vi "MDAQ_Main.vi"() -> ()   [LabVIEW 2021]
uses:
  FunctionVIS/Status_Def.ctl
  FunctionVIS/GUI_Def.ctl
  FunctionVIS/Mode_Enum.ctl
  FunctionVIS/Status_Cluster.ctl
  FunctionVIS/Array_Cluster.ctl
  FunctionVIS/CMD_ARG_Enum.ctl
  FunctionVIS/ARG_Cluster.ctl
  <vilib>/Analysis/1siggen.llb/Ramp Pattern by Samples.vi
  <vilib>/Analysis/NI_AALBase.lvlib
panel:
  in  "Tab Control 2":T1(tab)
  out "MDAQ Monitor":string
  in  "Clear_Monitor_Button":bool
  in  "Print_Help_Button":bool
  in  "Load_Button":bool
  in  "Save_Button":bool
  in  "Clear_Button":bool
  out "Collecting":bool
  in  "StartAq_Button":bool
  out "Waveform Graph":u32[](graph)
  in  "Get_Button":bool
  in  "StopAq_Button":bool
  out "Progress":u8(slide) scale=0.0..30.0
  in  "ForceW_Button":bool
  in  "Tab Control 3":T2(tab)
  out "XY Graph":T3(graph)
  in  "Save_CV_Button":bool
  out "Temp Graph":T4(graph)
  in  "Save_CV_Button 2":bool
  out "Amplitude Plot":cluster{"X":dbl, "Y":dbl}[](graph)
  out "CurrectSpectrum":u32[](graph)
  out "Surface CV Plot":dbl[][](graph)
  out "Collecting CV":bool
  in  "StartCV_Button":bool
  in  "StopCV_Button":bool
  out "CV-Prog":u8(slide) scale=0.0..1.0
  in  "Tab Control 4":T5(tab)
  in  "Update_Cal_Button":bool
  in  "Stop":bool
  in  "Tab Control":T6(tab)
  out "Temp B (K)":dbl
  out "Temp A (K)":dbl
  in  "Call_LS335":bool
  in  "Reset_Button":bool
  in  "Channels":T7(radio)=enum."Item 1"
  in  "Wave Form":enum32{"Item 0", "Item 1", "Radio Selection 3"}(radio)=enum."Item 1"
  in  "Send_Button":bool
  in  "Gate Stop":dbl=87.5 min=0.0 max=100.0 format="%.1f%%"
  in  "Gate Start":dbl=12.5 min=0.0 max=100.0 format="%.1f%%"
  in  "Amplitude":dbl min=0.0 max=16383.0 step=1.0
  in  "Frequency":dbl=10.0 min=1.0 max=114.0 step=0.05 format="%.2g"
  out "LakeShore?":bool
  in  "User Comments":string="Enter Comments here!"
  in  "Sample Name":string="Default Name"
  in  "CV Mode":enum32{"Item 0", "Item 1"}(radio)
  out "Elapsed Time":dbl format="%<%H:%M>t"
  in  "Master File Path":path
  out "Current Scan No.":i32
  in  "SendRamp_Button":bool
  in  "Steps":dbl=1.0 min=1.0 max=16383.0 step=1.0 format="%#.0f"
  in  "End":dbl min=0.0 max=16383.0 step=1.0 format="%#.0f"
  in  "Start":dbl min=0.0 max=16383.0 step=1.0 format="%#.0f"
  in  "Normalise Graph":bool
  out "Current Index":u32
  out "Delta T per Cycle (s)":dbl
  out "Target Values":i32
  in  "Refresh CV":bool
  in  "Target Bins/Ampl":dbl[](array[numeric]) min=0.0 max=16383.0 step=1.0
  in  "Delta T (s)":dbl=30.0
  in  "Manual_Send":bool
  in  "String":string
  out "error out":errorcluster {"code" format="%.0x"}
  in  "MDAQ209B COM Port":refnum<visa-resource-name>="COM4"
  # "Regular"
  # "Mirror"
  # "Index 0 is the value used for normalisation"
  # "Min:  0\nZero: \nMax: 16383"
  # "WARNING! Only use this function if you understand how the text\ncommands of the MDAQ works. Failure to do so may freeze the MDAQ\nand require you to power cylce the device. You have been warned."
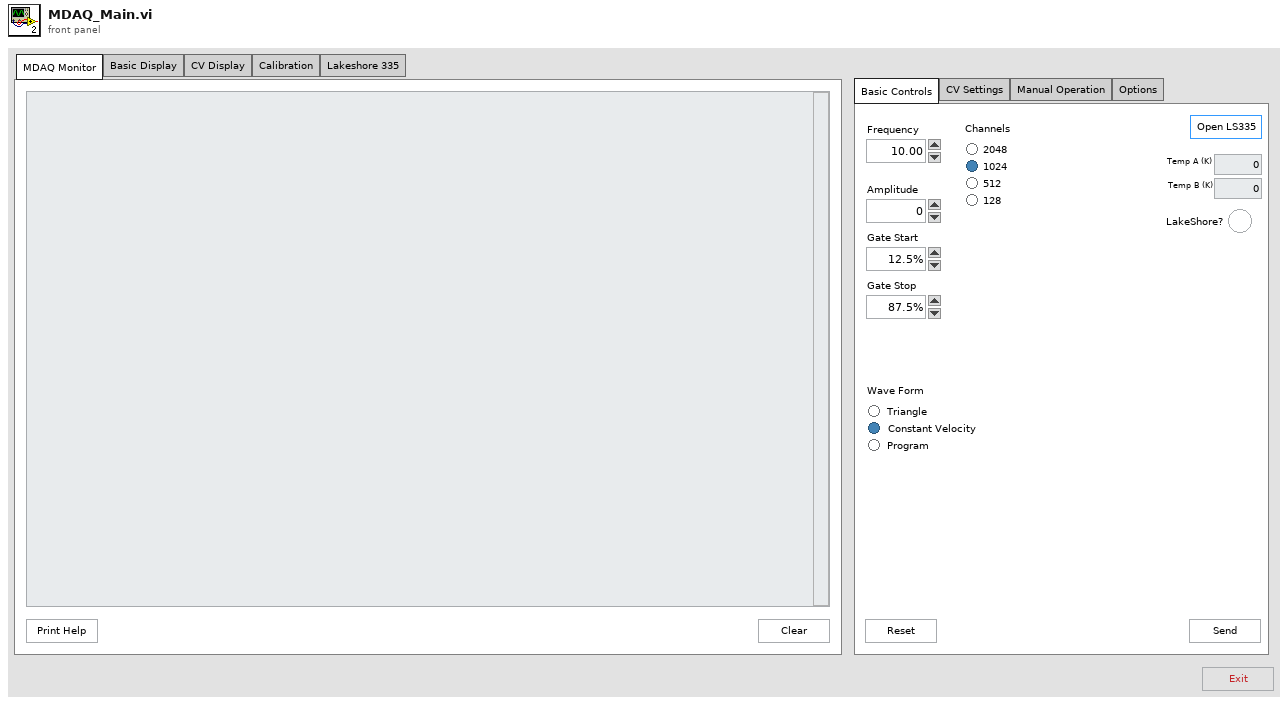
[diagram p1: front panel]
types:
  T1 = enum32{"MDAQ Monitor", "Basic Display", "CV Display", "Calibration", "Lakeshore 335"}
  T2 = enum32{"Time Plot", "Temperature Plot", "Amplitude Plot", "Current Spectrum", "Surface CV Plot"}
  T3 = cluster{"SetPointArray":cluster{timestamp, dbl}[]}[]
  T4 = cluster{"Counts Array":cluster{"Avg Temp":dbl, dbl}[]}[]
  T5 = enum32{"Spectrum Selection", "Calibration Overview"}
  T6 = enum32{"Basic Controls", "CV Settings", "Manual Operation", "Options"}
  T7 = enum32{"Item 0", "Item 1", "Radio Selection 3", ""}
  T8 = enum8{"Enabled", "Disabled", "Disabled and Grayed Out"}
  T9 = typedef "Status_Def.ctl" = enum16{"ClearCVCycle", "WriteCVData", "SendRamp", "LoadSpectrum", "RefreshCV", "SaveCVPlot", "GetCVSpectrum", "ConfigCV", "StopCV", "StartCV", "SaveSpectrum", "Clear Spectrum", "StopCollecting", "StopAq", "StartAq", "Reset MDAQ", "Get Spectrum", "Clear Monitor", "Idle", "String Send", "Settings Send", "Read Help"}
  T10 = typedef "Array_Cluster.ctl" = cluster{"CV Data Array":cluster{"Counts Array":cluster{timestamp, i32}[]}[], "CV Normalised Array":cluster{"Counts Array":cluster{timestamp, dbl}[]}[], "CV Temp Array":cluster{"Counts Array":cluster{"Avg Temp":dbl, dbl}[]}[]}
  T11 = typedef "Status_Cluster.ctl" = cluster{"CHAN":u32, "BASE":u32, "STEP":u32, "N_CYCLES":u32, "M_CYCLES":u32, "AMPLITUDE":u32, "GATESTRT":u32, "GATESTOP":u32, "Spectrum Array":u32[], "Spectrum Cycle":u32[][], "Cycle Timestamps":timestamp[], "Temperature Collect":dbl[]}
  T12 = typedef "GUI_Def.ctl" = cluster{"Monitor MSG":string, "Request Read":bool, "Cycle TimeStamp":timestamp, "CV":cluster{"Set Point Index":u32, "Run Start TimeS":timestamp, "Last SP Index":u32, "No. Set Points":u32, "Target Set Points":i32[], "Reverse?":bool, "NormalizationFactor":i32[], "CycleNo":i32, "SurfaceCV":dbl[][], "New Cycle":bool, "Temperature Array":dbl[][]}, "Normal":cluster{"Collecting":bool}, "Getting Mode":T13}
  T13 = typedef "Mode_Enum.ctl" = enum16{"Off", "Normal", "CV+Temp", "CV"}
  T14 = typedef "CMD_ARG_Enum.ctl" = enum16{"N_Cycles", "GateStep", "ASCII_Spectrum", "Waveform", "GateStop", "GateStart", "Amplitude", "Frequency"}
  T15 = typedef "ARG_Cluster.ctl" = cluster{"Freq":dbl, "Amp":dbl, "Chan Start":dbl, "Chan End":dbl, "Wave Form":enum32{"Item 0", "Item 1", "Radio Selection 3"}, "Channels":enum32{"Item 0", "Item 1", "Radio Selection 3", ""}}
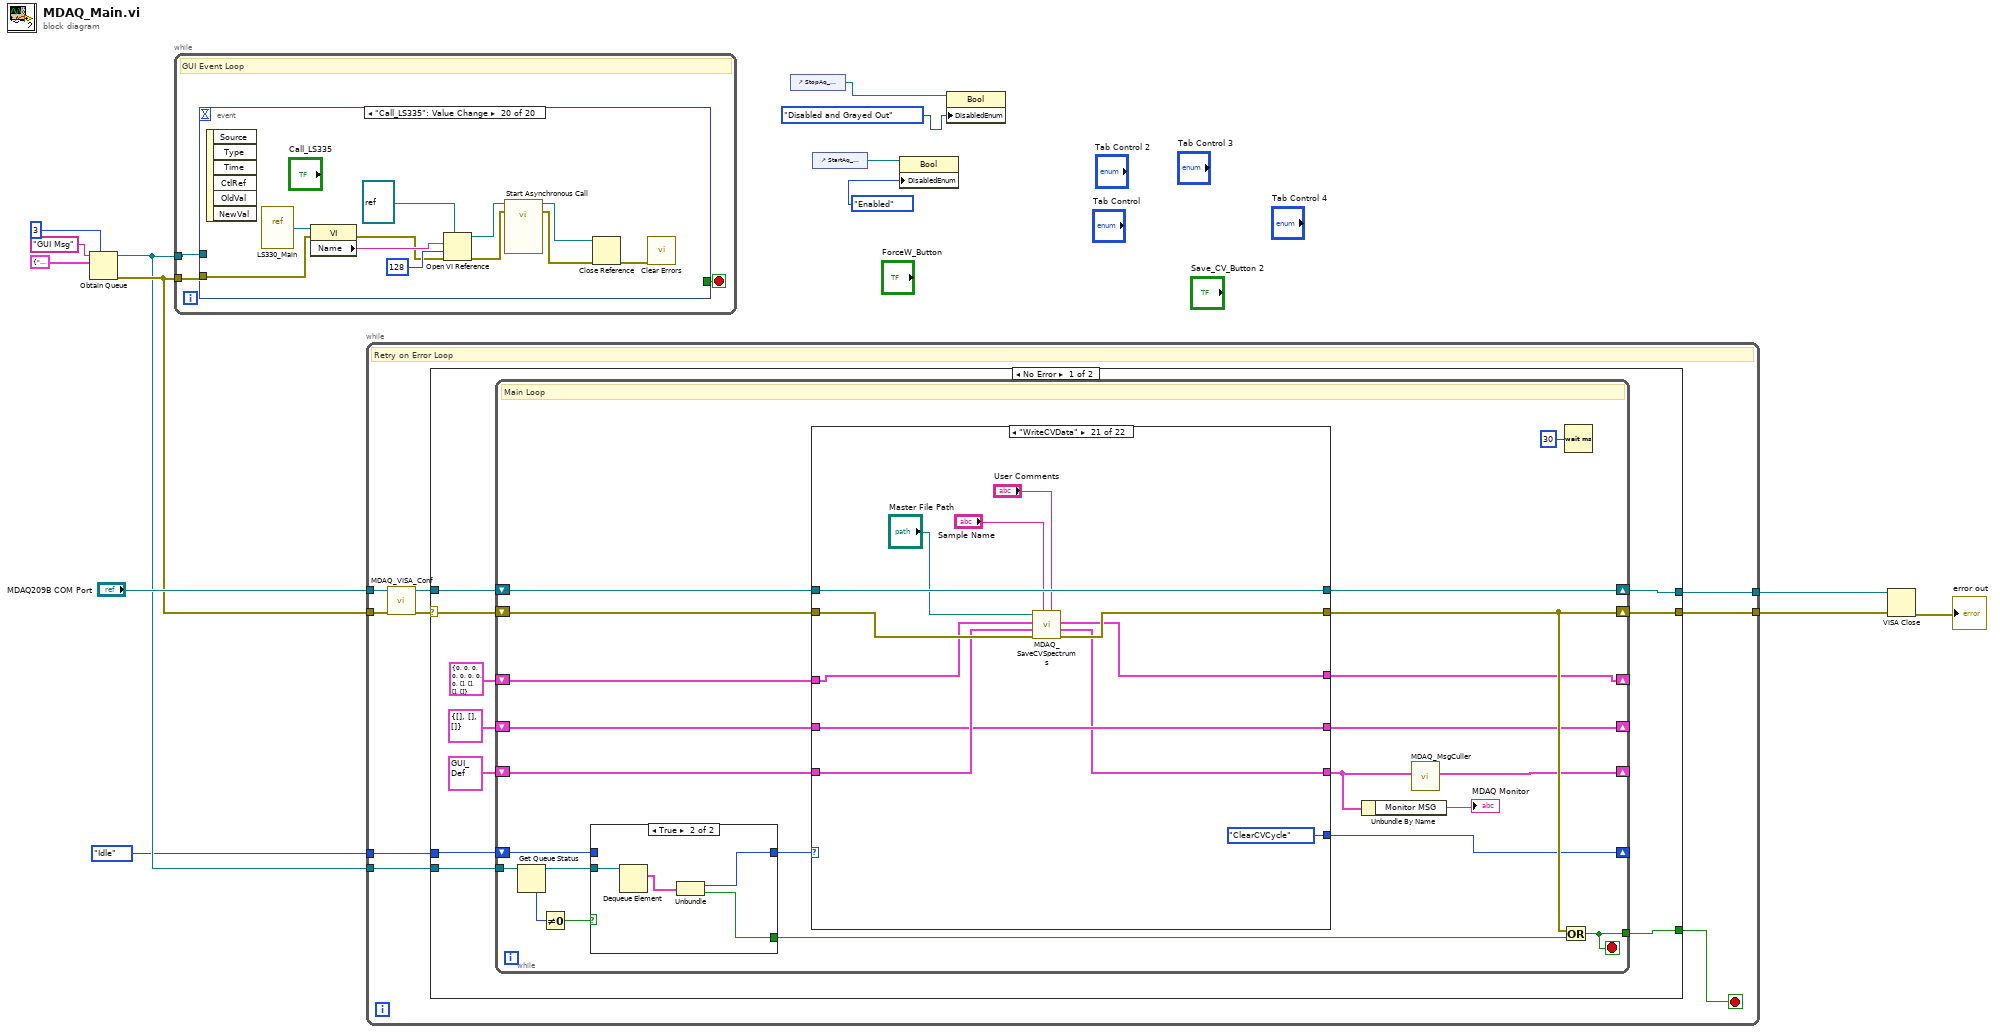
[diagram p0: block diagram]
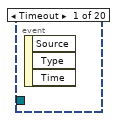
[diagram p2: hidden frame]
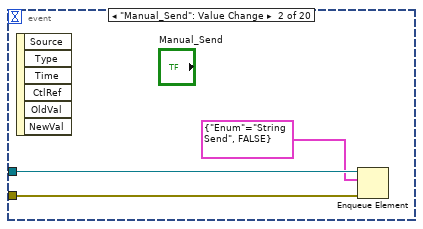
[diagram p3: hidden frame]
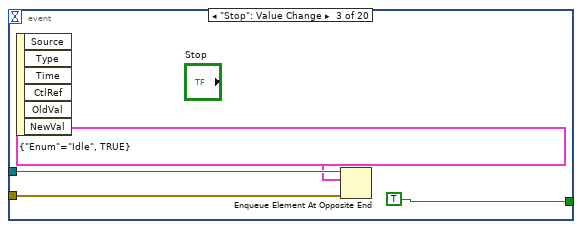
[diagram p4: hidden frame]
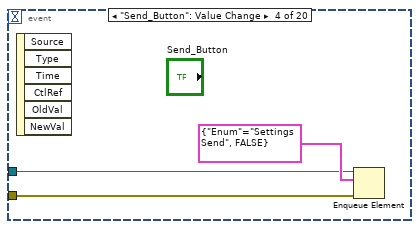
[diagram p5: hidden frame]
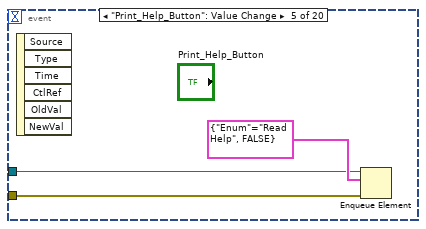
[diagram p6: hidden frame]
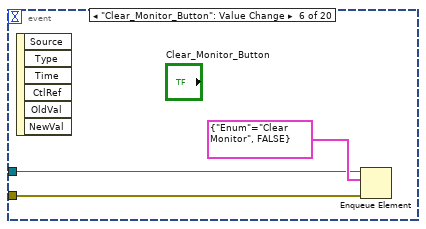
[diagram p7: hidden frame]
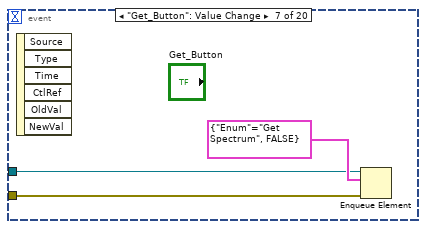
[diagram p8: hidden frame]
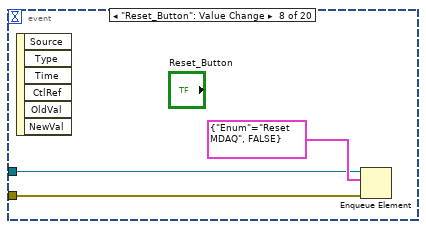
[diagram p9: hidden frame]
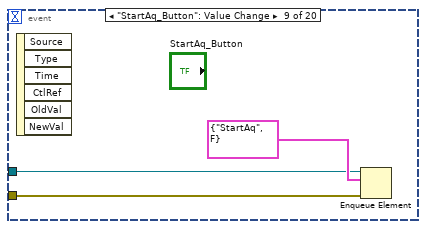
[diagram p10: hidden frame]
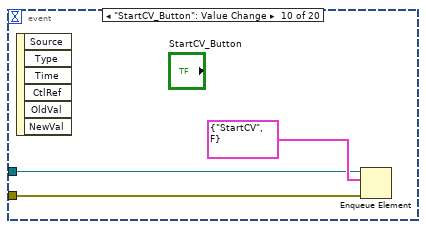
[diagram p11: hidden frame]
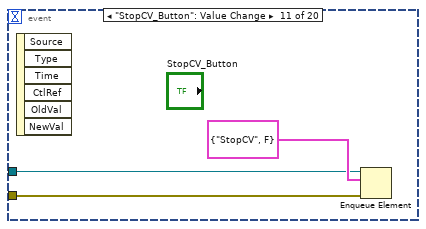
[diagram p12: hidden frame]
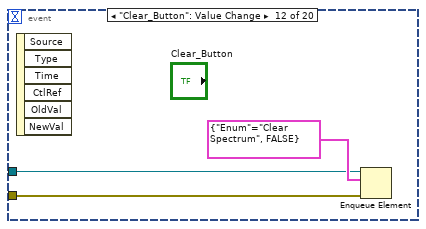
[diagram p13: hidden frame]
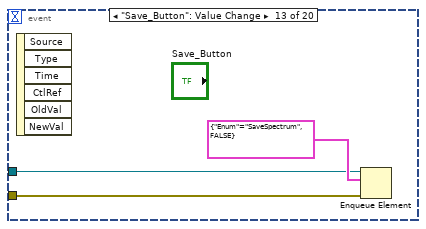
[diagram p14: hidden frame]
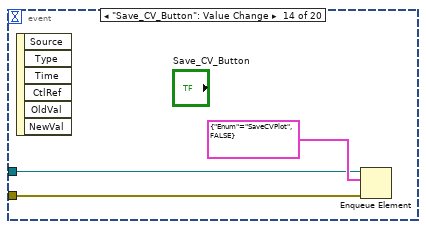
[diagram p15: hidden frame]
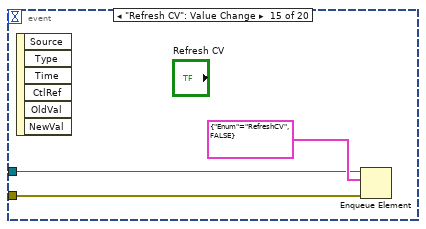
[diagram p16: hidden frame]
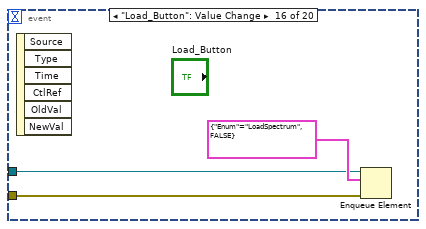
[diagram p17: hidden frame]
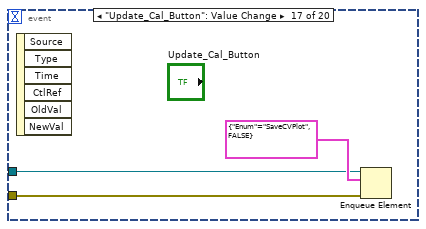
[diagram p18: hidden frame]
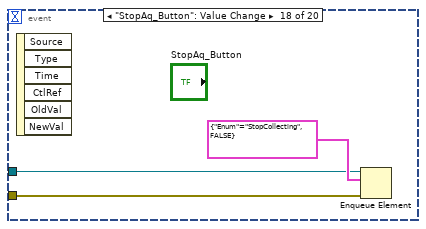
[diagram p19: hidden frame]
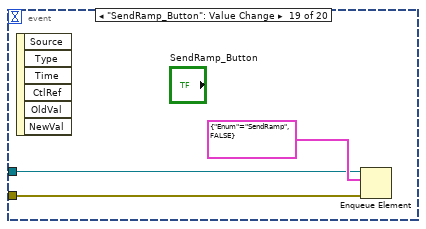
[diagram p20: hidden frame]
diagram:
  n1 = Obtain Queue(max queue size (-1, unlimited)=3, name (unnamed)="GUI Msg", element data type=cluster{"Enum":T9, bool} {"Enum"=enum."Read Help", TRUE}) -> (queue out=w9:refnum<queue>, error out=w10:errorcluster)  [unwired: 2 in, 1 out]
  n2 = while {
    tunnel: w10 -> [w17]
    tunnel: w9 -> [w16]
    stop <- w15 stop-if-true
    # "GUI Event Loop"
    n3 = event shown="[19] \"Call_LS335\": Value Change" {
      selector: _ -> [_ _ _ _ _ _ _ _ _ _ _ _ _ _ _ _ _ _ _ _]
      dyn-events: _ -> [_ _ _ _ _ _ _ _ _ _ _ _ _ _ _ _ _ _ _ _]
      timeout: _ -> [_ _ _ _ _ _ _ _ _ _ _ _ _ _ _ _ _ _ _ _]
      tunnel: w16 -> [_ w20 w24 w26 w29 w32 w35 w38 w41 w44 w47 w50 w53 w56 w59 w62 w65 w68 w71 _]
      tunnel: w17 -> [_ w18 w23 w25 w28 w31 w34 w37 w40 w43 w46 w49 w52 w55 w58 w61 w64 w67 w70 w80]
      tunnel: [_ _ TRUE _ _ _ _ _ _ _ _ _ _ _ _ _ _ _ _ _] -> w15
      event Timeout {
        n4 = event-data() -> ()  [unwired: 1 in, 3 out]
      }
      event "Manual_Send": Value Change {
        n5 = event-data() -> ()  [unwired: 1 in, 6 out]
        n6 = Enqueue Element(queue=w20, element=cluster{"Enum":T9, bool} {"Enum"=enum."String Send", FALSE}, error in (no error)=w18) -> ()  [unwired: 1 in, 3 out]
      }
      event "Stop": Value Change {
        n7 = event-data() -> ()  [unwired: 1 in, 6 out]
        n8 = Enqueue Element At Opposite End(queue=w24, element=cluster{"Enum":T9, bool} {"Enum"=enum."Idle", TRUE}, error in (no error)=w23) -> ()  [unwired: 1 in, 3 out]
      }
      event "Send_Button": Value Change {
        n9 = event-data() -> ()  [unwired: 1 in, 6 out]
        n10 = Enqueue Element(queue=w26, element=cluster{"Enum":T9, bool} {"Enum"=enum."Settings Send", FALSE}, error in (no error)=w25) -> ()  [unwired: 1 in, 3 out]
      }
      event "Print_Help_Button": Value Change {
        n11 = event-data() -> ()  [unwired: 1 in, 6 out]
        n12 = Enqueue Element(queue=w29, element=cluster{"Enum":T9, bool} {"Enum"=enum."Read Help", FALSE}, error in (no error)=w28) -> ()  [unwired: 1 in, 3 out]
      }
      event "Clear_Monitor_Button": Value Change {
        n13 = event-data() -> ()  [unwired: 1 in, 6 out]
        n14 = Enqueue Element(queue=w32, element=cluster{"Enum":T9, bool} {"Enum"=enum."Clear Monitor", FALSE}, error in (no error)=w31) -> ()  [unwired: 1 in, 3 out]
      }
      event "Get_Button": Value Change {
        n15 = event-data() -> ()  [unwired: 1 in, 6 out]
        n16 = Enqueue Element(queue=w35, element=cluster{"Enum":T9, bool} {"Enum"=enum."Get Spectrum", FALSE}, error in (no error)=w34) -> ()  [unwired: 1 in, 3 out]
      }
      event "Reset_Button": Value Change {
        n17 = event-data() -> ()  [unwired: 1 in, 6 out]
        n18 = Enqueue Element(queue=w38, element=cluster{"Enum":T9, bool} {"Enum"=enum."Reset MDAQ", FALSE}, error in (no error)=w37) -> ()  [unwired: 1 in, 3 out]
      }
      event "StartAq_Button": Value Change {
        n19 = event-data() -> ()  [unwired: 1 in, 6 out]
        n20 = Enqueue Element(queue=w41, element=cluster{"Enum":T9, bool} {"Enum"=enum."StartAq", FALSE}, error in (no error)=w40) -> ()  [unwired: 1 in, 3 out]
      }
      event "StartCV_Button": Value Change {
        n21 = event-data() -> ()  [unwired: 1 in, 6 out]
        n22 = Enqueue Element(queue=w44, element=cluster{"Enum":T9, bool} {"Enum"=enum."StartCV", FALSE}, error in (no error)=w43) -> ()  [unwired: 1 in, 3 out]
      }
      event "StopCV_Button": Value Change {
        n23 = event-data() -> ()  [unwired: 1 in, 6 out]
        n24 = Enqueue Element(queue=w47, element=cluster{"Enum":T9, bool} {"Enum"=enum."StopCV", FALSE}, error in (no error)=w46) -> ()  [unwired: 1 in, 3 out]
      }
      event "Clear_Button": Value Change {
        n25 = event-data() -> ()  [unwired: 1 in, 6 out]
        n26 = Enqueue Element(queue=w50, element=cluster{"Enum":T9, bool} {"Enum"=enum."Clear Spectrum", FALSE}, error in (no error)=w49) -> ()  [unwired: 1 in, 3 out]
      }
      event "Save_Button": Value Change {
        n27 = event-data() -> ()  [unwired: 1 in, 6 out]
        n28 = Enqueue Element(queue=w53, element=cluster{"Enum":T9, bool} {"Enum"=enum."SaveSpectrum", FALSE}, error in (no error)=w52) -> ()  [unwired: 1 in, 3 out]
      }
      event "Save_CV_Button": Value Change {
        n29 = event-data() -> ()  [unwired: 1 in, 6 out]
        n30 = Enqueue Element(queue=w56, element=cluster{"Enum":T9, bool} {"Enum"=enum."SaveCVPlot", FALSE}, error in (no error)=w55) -> ()  [unwired: 1 in, 3 out]
      }
      event "Refresh CV": Value Change {
        n31 = event-data() -> ()  [unwired: 1 in, 6 out]
        n32 = Enqueue Element(queue=w59, element=cluster{"Enum":T9, bool} {"Enum"=enum."RefreshCV", FALSE}, error in (no error)=w58) -> ()  [unwired: 1 in, 3 out]
      }
      event "Load_Button": Value Change {
        n33 = event-data() -> ()  [unwired: 1 in, 6 out]
        n34 = Enqueue Element(queue=w62, element=cluster{"Enum":T9, bool} {"Enum"=enum."LoadSpectrum", FALSE}, error in (no error)=w61) -> ()  [unwired: 1 in, 3 out]
      }
      event "Update_Cal_Button": Value Change {
        n35 = event-data() -> ()  [unwired: 1 in, 6 out]
        n36 = Enqueue Element(queue=w65, element=cluster{"Enum":T9, bool} {"Enum"=enum."SaveCVPlot", FALSE}, error in (no error)=w64) -> ()  [unwired: 1 in, 3 out]
      }
      event "StopAq_Button": Value Change {
        n37 = event-data() -> ()  [unwired: 1 in, 6 out]
        n38 = Enqueue Element(queue=w68, element=cluster{"Enum":T9, bool} {"Enum"=enum."StopCollecting", FALSE}, error in (no error)=w67) -> ()  [unwired: 1 in, 3 out]
      }
      event "SendRamp_Button": Value Change {
        n39 = event-data() -> ()  [unwired: 1 in, 6 out]
        n40 = Enqueue Element(queue=w71, element=cluster{"Enum":T9, bool} {"Enum"=enum."SendRamp", FALSE}, error in (no error)=w70) -> ()  [unwired: 1 in, 3 out]
      }
      event "Call_LS335": Value Change {
        n41 = event-data() -> ()  [unwired: 1 in, 6 out]
        n42 = vi-ref "LS330_Main.vi"() -> (w83:refnum<vi>)
        n43 = property class="VI"(reference=w83, error in=w80) -> (error out=w79:errorcluster, "Name"=w82:string)  [unwired: 1 out]
        n44 = Open VI Reference(type specifier VI Refnum (for type only)=refnum<vi> refnum, vi path=w82, options=128, error in (no error)=w79) -> (vi reference=w76:refnum<vi>, error out=w78:errorcluster)  [unwired: 2 in]
        n45 = call-by-ref "Start Asynchronous Call"(reference=w76, error in=w78) -> (reference out=w75:refnum<vi>, error out=w74:errorcluster)  [unwired: 12 in]
        n46 = Close Reference(reference=w75, error in (no error)=w74) -> (error out=w73:errorcluster)
        n47 = call <vilib>:"Clear Errors.vi"("error in (no error)"=w73) -> ()  [unwired: 5 in, 2 out]
      }
    }
  }
  n48 = while {
    tunnel: "MDAQ209B COM Port" -> [w92]
    tunnel: w10 -> [w90]
    tunnel: w9 -> [w88]
    tunnel: [w87] -> w7
    tunnel: [w86] -> w8
    tunnel: Status_Def."Idle" ("Enum") -> [w84]
    stop <- w85 stop-if-true
    # "Retry on Error Loop"
    n49 = call "MDAQ_VISA_Conf.vi"("error in"=w90, "VISA resource name"=w92) -> ("error out"=w91:errorcluster, "VISA resource name out"=w89:refnum<visa-resource-name>)  [unwired: 8 in]
    n50 = case shown="No Error" w91 {
      selector: w91 -> [w100 w596]
      tunnel: w89 -> [w101 w597]
      tunnel: w88 -> [w102 _]
      tunnel: [w99 w596] -> w87
      tunnel: [w98 w597] -> w86
      tunnel: [w97 TRUE] -> w85
      tunnel: w84 -> [w96 _]
      frame No Error {
        n51 = while {
          tunnel: w102 -> [w121]
          shift-right: [w117] -> w98
          shift-left: w101 -> [w119]
          shift-right: [w116] -> w99
          shift-left: w100 -> [w118]
          shift-right: [w103] -> _
          shift-left: T12 {"Monitor MSG"="", "Request Read"=FALSE, "Cycle TimeStamp"=timestamp(0 s since 1904-01-01), "CV"={"Set Point Index"=0, "Run Start TimeS"=timestamp(0 s since 1904-01-01), "Last SP Index"=0, "No. Set Points"=0, "Target Set Points"=[], "Reverse?"=FALSE, "NormalizationFactor"=[], "CycleNo"=0, "SurfaceCV"=[], "New Cycle"=FALSE, "Temperature Array"=[]}, "Normal"={"Collecting"=FALSE}, "Getting Mode"=enum."Off"} ("Main Cluster") -> [w110]
          tunnel: [w114] -> w97
          shift-right: [w111] -> _
          shift-left: w96 -> [w112]
          shift-right: [w107] -> _
          shift-left: T11 {"CHAN"=0, "BASE"=0, "STEP"=0, "N_CYCLES"=0, "M_CYCLES"=0, "AMPLITUDE"=0, "GATESTRT"=0, "GATESTOP"=0, "Spectrum Array"=[], "Spectrum Cycle"=[], "Cycle Timestamps"=[], "Temperature Collect"=[]} ("Status Cluster") -> [w108]
          shift-right: [w106] -> _
          shift-left: T10 {"CV Data Array"=[], "CV Normalised Array"=[], "CV Temp Array"=[]} ("Concurrent CV Arrays") -> [w105]
          stop <- w114 stop-if-true
          # "Main Loop"
          n52 = Get Queue Status(queue=w121) -> (queue out=w122:refnum<queue>, # elements in queue=w123:i32)  [unwired: 2 in, 6 out]
          n53 = Not Equal To 0?(x=w123) -> (x != 0?=w124:bool)
          n54 = case shown="True" w124 {
            tunnel: w122 -> [_ w130]
            tunnel: w112 -> [w126 _]
            tunnel: [w126 w128] -> w120
            tunnel: [FALSE w127] -> w115
            frame False {
            }
            frame True {
              n55 = Dequeue Element(queue=w130) -> (element=w129:cluster{"Enum":T9, bool})  [unwired: 2 in, 3 out]
              n56 = Unbundle(w129) -> ("Enum"=w128:T9, w127:bool)
            }
          }
          n57 = case shown="\"WriteCVData\"" w120 {
            selector: w120 -> [w139 _ _ _ _ _ _ _ _ _ _ _ _ _ _ _ _ _ _ _ _ _]
            tunnel: [w136 Status_Def."Idle" ("Enum") Status_Def."Idle" ("Enum") w221 Status_Def."Idle" ("Enum") Status_Def."ConfigCV" ("Enum") Status_Def."Idle" ("Enum") w327 Status_Def."Idle" ("Enum") Status_Def."Idle" ("Enum") w384 w429 Status_Def."Idle" ("Enum") Status_Def."Idle" ("Enum") Status_Def."Idle" ("Enum") Status_Def."Idle" ("Enum") w524 w545 Status_Def."Idle" ("Enum") Status_Def."Idle" ("Enum") Status_Def."ClearCVCycle" ("Enum") Status_Def."Idle" ("Enum")] -> w111
            tunnel: w119 -> [w146 w201 w212 w233 w247 w283 w312 w340 w355 w360 w382 w435 w476 w488 w492 w501 w536 w543 w561 w567 w580 w588]
            tunnel: w118 -> [w145 w200 w211 w232 w246 w282 w311 w337 w354 w359 w381 w434 w458 w487 w491 w499 w535 w542 w557 w563 w577 w587]
            tunnel: [w148 w197 w208 w231 w248 w280 w309 w342 w354 w357 w379 w423 w457 w486 w491 w504 w527 w544 w556 w565 w574 w587] -> w116
            tunnel: [w147 w198 w209 w230 w249 w281 w310 w343 w355 w358 w380 w424 w476 w485 w492 w505 w528 w543 w561 w567 w580 w588] -> w117
            tunnel: [w142 w204 w216 w228 w259 w267 w302 w322 w352 w370 w385 w406 w462 w481 w494 w514 w533 w551 w560 w564 w571 w584] -> w104
            tunnel: w110 -> [w135 w206 w218 w229 w261 w289 w301 w331 w352 w372 w376 w427 w467 w483 w496 w515 w526 w549 w560 w564 w575 w585]
            tunnel: w108 -> [w133 w203 w215 w227 w258 w273 w299 w339 w353 w369 w378 w433 w475 w480 w493 w500 w534 w541 w558 w566 w576 w583]
            tunnel: [w132 w203 w215 w227 w258 w272 w299 w324 w353 w369 w377 w407 w475 w480 w493 w503 w519 w541 w555 w566 w572 w582] -> w107
            tunnel: [w131 w202 w214 w220 w250 w266 w293 w313 w345 w356 w374 w401 w456 w478 w489 w498 w517 w539 w552 w562 w573 w581] -> w106
            tunnel: w105 -> [w131 w202 w214 w220 w250 w265 w293 w313 w345 w356 w374 w402 w456 w478 w489 w498 w517 w539 w552 w562 w573 w581]
            frame "Idle", Default {
              n58 = Unbundle By Name(w135) -> ("Monitor MSG"=w144:string, "Request Read"=w143:bool, "Cycle TimeStamp"=w137:timestamp, "Getting Mode"=w138:T13)
              n59 = case shown="False" w143 {
                tunnel: w145 -> [w186 w194]
                tunnel: [w186 w192] -> w148
                tunnel: [w187 w193] -> w147
                tunnel: w146 -> [w187 w195]
                tunnel: [FALSE w191] -> w141
                tunnel: w144 -> [w184 w190]
                tunnel: [w184 w188] -> w140
                frame False {
                }
                frame True {
                  n60 = call "MDAQ_ReadAll.vi"("error in"=w194, "VISA resource name"=w195) -> ("error IO"=w192:errorcluster, "Buffer Not Empty"=w191:bool, "read buffer"=w189:string, "VISA resource name out"=w193:refnum<visa-resource-name>)  [unwired: 6 in]
                  n61 = Concatenate Strings(w190, w189) -> (w188:string)
                }
              }
              n62 = case shown="\"CV+Temp\"" w138 {
                tunnel: w139 -> [w150 w158 w168 w179]
                tunnel: w137 -> [_ w161 _ _]
                tunnel: [w150 w154 w164 w178] -> w136
                tunnel: w135 -> [w151 w153 w167 w180]
                tunnel: [w151 w153 w166 w177] -> w134
                tunnel: w133 -> [w149 w152 w163 w176]
                tunnel: [w149 w152 w163 w175] -> w132
                frame "Off", Default {
                }
                frame "Normal" {
                  (unwired) 0.0
                  n63 = Get Date/Time In Seconds() -> (seconds since 1Jan1904=w162:timestamp)
                  n64 = Subtract(x=w162, y=w161) -> (x-y=w155:dbl)
                  n65 = Greater Or Equal?(x=w155, y=30.0) -> (x >= y?=w159:bool)
                  n66 = To Unsigned Byte Integer(number=w155) -> (unsigned 8bit integer=→"Progress":u8)
                  n67 = Select(t=Status_Def."StopAq", s=w159, f=w158) -> (s? t:f=w154:T9)
                }
                frame "CV" {
                  # "Idle"
                  # "StopAq"
                  n68 = control-ref of="CV-Prog"() -> (w171:refnum<vi>)
                  n69 = call "MDAQ_KeepTime.vi"("Delta T (s)"="Delta T (s)", "State in"=w168, "Cluster In"=w167, "Slide in"=w171) -> ("State Out"=w164:T9, "Cluster Out"=w166:T12, "Progress"=→"CV-Prog":u8, "Elapsed Out"=→"Elapsed Time":dbl)  [unwired: 4 in]
                }
                frame "CV+Temp" {
                  # "Idle"
                  # "StopAq?"
                  n70 = control-ref of="Elapsed Time"() -> (w181:refnum<vi>)
                  n71 = control-ref of="CV-Prog"() -> (w183:refnum<vi>)
                  n72 = control-ref of="Delta T (s)"() -> (w182:refnum<vi>)
                  n73 = call "MDAQ_GetTimeTemp.vi"("Elapsed Time Ref"=w181, "Delta T (s) Ref"=w182, "State in"=w179, "Cluster In"=w180, "Status In"=w176, "CV-Prog Ref"=w183) -> ("State Out"=w178:T9, "Cluster Out"=w177:T12, "Status Out"=w175:T11, "Temps"=w174:cluster{"Double":dbl, "Double":dbl})  [unwired: 2 in]
                  n74 = Unbundle(w174) -> ("Double"=→"Temp A (K)":dbl, "Double"=→"Temp B (K)":dbl)
                }
              }
              n75 = Bundle By Name(cluster=w134, "Monitor MSG"=w140, "Request Read"=w141) -> (w142:T12)
            }
            frame "String Send" {
              n76 = call "MDAQ_WRITE.vi"("error in"=w200, "ARG"="", "CMD"="String", "VISA resource name"=w201) -> ("error out"=w197:errorcluster, "VISA resource name out"=w198:refnum<visa-resource-name>)  [unwired: 6 in]
              n77 = Bundle By Name(cluster=w206, "Request Read"=TRUE) -> (w204:T12)
            }
            frame "Reset MDAQ" {
              n78 = call "MDAQ_WRITE.vi"("error in"=w211, "ARG"="", "CMD"="R" ("write buffer"), "VISA resource name"=w212) -> ("error out"=w208:errorcluster, "VISA resource name out"=w209:refnum<visa-resource-name>)  [unwired: 6 in]
              n79 = Bundle By Name(cluster=w218, "Request Read"=TRUE) -> (w216:T12)
            }
            frame "Clear Spectrum" {
              n80 = Two Button Dialog(message="Are you sure you want to clear the MDAQ spectrum buffer?", 1:"No" ("F button name (\"Cancel\")"), 2:"Yes" ("T button name (\"OK\")")) -> (T button?=w225:bool)
              n81 = case shown="True" w225 {
                tunnel: w233 -> [w239 w243]
                tunnel: w232 -> [w238 w242]
                tunnel: [w236 w242] -> w231
                tunnel: [w237 w243] -> w230
                tunnel: [TRUE FALSE] -> w226
                tunnel: [Status_Def."Get Spectrum" ("Enum") Status_Def."Idle" ("Enum")] -> w221
                frame True {
                  n82 = call "MDAQ_WRITE.vi"("error in"=w238, "ARG"="", "CMD"="Z" ("write buffer"), "VISA resource name"=w239) -> ("error out"=w236:errorcluster, "VISA resource name out"=w237:refnum<visa-resource-name>)  [unwired: 6 in]
                }
                frame False {
                }
              }
              n83 = Bundle By Name(cluster=w229, "Request Read"=w226) -> (w228:T12)
            }
            frame "StartAq" {
              n84 = control-ref of="StopAq_Button"() -> (w253:refnum<vi>)
              n85 = control-ref of="StartAq_Button"() -> (w255:refnum<vi>)
              n86 = property class="Bool"(reference=w253, "DisabledEnum"=T8."Enabled" ("Disabled")) -> ()  [unwired: 1 in, 2 out]
              n87 = property class="Bool"(reference=w255, "DisabledEnum"=T8."Disabled and Grayed Out" ("Disabled")) -> ()  [unwired: 1 in, 2 out]
              n88 = call "MDAQ_StartAq.vi"("error in (no error)"=w246, "VISA Refnum in"=w247) -> ("error out"=w248:errorcluster, "VISA Refnum out"=w249:refnum<visa-resource-name>)  [unwired: 8 in]
              n89 = Get Date/Time In Seconds() -> (seconds since 1Jan1904=w257:timestamp)
              n90 = Bundle By Name(cluster=w261, "Getting Mode"=Mode_Enum."Normal", "Request Read"=TRUE, "Cycle TimeStamp"=w257) -> (w259:T12)
              "Collecting" <- TRUE ("Collecting")
            }
            frame "StartCV" {
              n91 = control-ref of="Target Bins/Ampl"() -> (w276:refnum<vi>)
              n92 = control-ref of="StartCV_Button"() -> (w279:refnum<vi>)
              n93 = control-ref of="Save_CV_Button"() -> (w278:refnum<vi>)
              n94 = case shown="\"Item 0\", Default" "CV Mode" {
                tunnel: [Mode_Enum."CV" ("Getting Mode") Mode_Enum."CV+Temp" ("Getting Mode")] -> w269
                frame "Item 0", Default {
                }
                frame "Item 1" {
                }
              }
              n95 = property class="Arr (strict)"(reference=w276) -> ("Value"=w263:dbl[])  [unwired: 1 in, 2 out]
              n96 = property class="Bool"(reference=w279, "DisabledEnum"=T8."Disabled and Grayed Out" ("Disabled")) -> ()  [unwired: 1 in, 2 out]
              n97 = property class="Bool"(reference=w278, "DisabledEnum"=T8."Disabled and Grayed Out" ("Disabled")) -> ()  [unwired: 1 in, 2 out]
              n98 = To Long Integer(number=w263) -> (32bit integer=w264:i32[])
              n99 = call "MDAQ_ClearSpec.vi"("error in (no error)"=w282, "VISA Refnum in"=w283) -> ("error out"=w280:errorcluster, "VISA Refnum out"=w281:refnum<visa-resource-name>)  [unwired: 8 in]
              n100 = Array Size(array=w263) -> (size(s)=w274:i32)
              n101 = Get Date/Time In Seconds() -> (seconds since 1Jan1904=w271:timestamp)
              n102 = control-ref of="StopCV_Button"() -> (w285:refnum<vi>)
              n103 = Bundle By Name(cluster=w289, "CV.Run Start TimeS"=w271, "CV.No. Set Points"=w274, "CV.Set Point Index"=u32 0, "CV.Target Set Points"=w264, "Getting Mode"=w269, "Request Read"=TRUE, "Cycle TimeStamp"=w271) -> (w268:T12)
              n104 = property class="Bool"(reference=w285, "DisabledEnum"=T8."Enabled" ("Disabled")) -> ()  [unwired: 1 in, 2 out]
              n105 = call "MDAQ_PrepCVArray.vi"("input cluster"=w268, "Concurrent CV Arrays"=w265, "Status_Cluster"=w273) -> ("Output cluster"=w267:T12, "Concurrent CV Arrays Out"=w266:T10, "Status_Cluster Out"=w272:T11)  [unwired: 6 in]
              "Collecting CV" <- TRUE ("Collecting")
            }
            frame "StopCV" {
              n106 = control-ref of="Save_CV_Button"() -> (w296:refnum<vi>)
              n107 = control-ref of="StartCV_Button"() -> (w305:refnum<vi>)
              n108 = control-ref of="StopCV_Button"() -> (w307:refnum<vi>)
              n109 = property class="Bool"(reference=w305, "DisabledEnum"=T8."Enabled" ("Disabled")) -> ()  [unwired: 1 in, 2 out]
              n110 = property class="Bool"(reference=w296, "DisabledEnum"=T8."Enabled" ("Disabled")) -> ()  [unwired: 1 in, 2 out]
              n111 = property class="Bool"(reference=w307, "DisabledEnum"=T8."Disabled and Grayed Out" ("Disabled")) -> ()  [unwired: 1 in, 2 out]
              n112 = call "MDAQ_StopAq.vi"("error in (no error)"=w311, "VISA Refnum in"=w312) -> ("error out"=w309:errorcluster, "VISA Refnum out"=w310:refnum<visa-resource-name>)  [unwired: 8 in]
              n113 = control-ref of="Collecting CV"() -> (w298:refnum<vi>)
              n114 = Get Date/Time In Seconds() -> (seconds since 1Jan1904=w303:timestamp)
              n115 = Bundle By Name(cluster=w301, "Getting Mode"=Mode_Enum."Off", "Request Read"=TRUE, "Cycle TimeStamp"=w303) -> (w302:T12)
              n116 = property class="Bool (strict)"(reference=w298, "Value"=FALSE) -> ()  [unwired: 1 in, 2 out]
            }
            frame "ConfigCV" {
              n117 = call "MDAQ_CMD_Write.vi"("CMD"=CMD_ARG_Enum."Waveform", "error in"=w337, "Status_Cluster"=w339, "ARG"=enum32{"Triangle", "CV", "Prog"}."CV" ("Wave Form"), "VISA resource name"=w340) -> ("error out"=w336:errorcluster, "Status_Cluster Out"=w338:T11, "VISA resource name out"=w333:refnum<visa-resource-name>)  [unwired: 4 in]
              n118 = call "MDAQ_IndexProgress.vi"("Input Cluster"=w331) -> ("output cluster"=w330:T12, "Selected Amplitude"=w332:dbl)  [unwired: 9 in]
              n119 = Get Date/Time In Seconds() -> (seconds since 1Jan1904=w341:timestamp)
              n120 = call "MDAQ_CMD_Write.vi"("CMD"=CMD_ARG_Enum."Amplitude", "error in"=w336, "Status_Cluster"=w338, "ARG"=w332, "VISA resource name"=w333) -> ("error out"=w317:errorcluster, "Status_Cluster Out"=w319:T11, "VISA resource name out"=w321:refnum<visa-resource-name>)  [unwired: 4 in]
              n121 = Unbundle By Name(w330) -> ("CV.Set Point Index"=→"Current Index":u32, "CV.New Cycle"=w326:bool)
              n122 = control-ref of="Frequency"() -> (w315:refnum<vi>)
              n123 = control-ref of="Delta T (s)"() -> (w314:refnum<vi>)
              n124 = Bundle By Name(cluster=w330, "Cycle TimeStamp"=w341) -> (w323:T12)
              n125 = call "MDAQ_SetCycleDelta.vi"("Delta T (s)"=w314, "Frequency"=w315, "error in"=w317, "Status_Cluster"=w319, "VISA resource name"=w321) -> ("error out"=w316:errorcluster, "Status_Cluster Out"=w318:T11, "VISA resource name out"=w320:refnum<visa-resource-name>)  [unwired: 4 in]
              n126 = call "MDAQ_SaveTime.vi"("Cluster In"=w323, "Status_Cluster"=w318) -> ("Cluster Out"=w322:T12, "Status_Cluster Out"=w324:T11)  [unwired: 8 in]
              n127 = call "MDAQ_StartAq.vi"("error in (no error)"=w316, "VISA Refnum in"=w320) -> ("error out"=w342:errorcluster, "VISA Refnum out"=w343:refnum<visa-resource-name>)  [unwired: 8 in]
              n128 = Select(t=Status_Def."WriteCVData", s=w326, f=Status_Def."Idle" ("Enum")) -> (s? t:f=w327:T9)
            }
            frame "SendRamp" {
              n129 = control-ref of="Target Bins/Ampl"() -> (w347:refnum<vi>)
              n130 = call-poly <vilib>:"Ramp Pattern.vi"("start"="Start", "end"="End", "samples"="Steps") -> ("Ramp Pattern"=w346:dbl[])  [unwired: 7 in, 1 out]
              n131 = property class="Arr (strict)"(reference=w347, "Value"=w346) -> ()  [unwired: 1 in, 2 out]
            }
            frame "StopCollecting" {
              n132 = control-ref of="StartAq_Button"() -> (w367:refnum<vi>)
              n133 = control-ref of="StopAq_Button"() -> (w365:refnum<vi>)
              n134 = property class="Bool"(reference=w367, "DisabledEnum"=T8."Enabled" ("Disabled")) -> ()  [unwired: 1 in, 2 out]
              n135 = property class="Bool"(reference=w365, "DisabledEnum"=T8."Disabled and Grayed Out" ("Disabled")) -> ()  [unwired: 1 in, 2 out]
              n136 = call "MDAQ_StopAq.vi"("error in (no error)"=w359, "VISA Refnum in"=w360) -> ("error out"=w357:errorcluster, "VISA Refnum out"=w358:refnum<visa-resource-name>)  [unwired: 8 in]
              n137 = control-ref of="Collecting"() -> (w363:refnum<vi>)
              n138 = Get Date/Time In Seconds() -> (seconds since 1Jan1904=w368:timestamp)
              n139 = property class="Bool (strict)"(reference=w363, "Value"=FALSE) -> ()  [unwired: 1 in, 2 out]
              n140 = Bundle By Name(cluster=w372, "Getting Mode"=Mode_Enum."Off", "Request Read"=TRUE, "Cycle TimeStamp"=w368) -> (w370:T12)
            }
            frame "StopAq" {
              n141 = Unbundle By Name(w376) -> ("Getting Mode"=w383:T13)
              n142 = case shown="\"CV+Temp\"" w383 {
                tunnel: [Status_Def."Idle" ("Enum") Status_Def."GetCVSpectrum" ("Enum") Status_Def."GetCVSpectrum" ("t") Status_Def."Get Spectrum" ("t")] -> w384
                tunnel: w378 -> [w388 w391 w396 w399]
                tunnel: [w388 w391 w394 w399] -> w377
                tunnel: w376 -> [w387 w390 w395 w398]
                tunnel: [w387 w390 w393 w398] -> w375
                frame "Off", Default {
                }
                frame "CV" {
                }
                frame "CV+Temp" {
                  n143 = call "MDAQ_CaptureTemps.vi"("Main Cluster"=w395, "Status Cluster"=w396) -> ("Main Cluster Out"=w393:T12, "Status Cluster Out"=w394:T11)  [unwired: 8 in]
                }
                frame "Normal" {
                }
              }
              n144 = call "MDAQ_StopAq.vi"("error in (no error)"=w381, "VISA Refnum in"=w382) -> ("error out"=w379:errorcluster, "VISA Refnum out"=w380:refnum<visa-resource-name>)  [unwired: 8 in]
              n145 = Bundle By Name(cluster=w375, "Request Read"=TRUE) -> (w385:T12)
            }
            frame "GetCVSpectrum" {
              n146 = Unbundle By Name(w427) -> ("Getting Mode"=w430:T13)
              n147 = control-ref of="CurrectSpectrum"() -> (w421:refnum<vi>)
              n148 = call "MDAQ_READ_Status.vi"("error in"=w434, "Status_Cluster IN"=w433, "VISA resource name"=w435) -> ("error out"=w437:errorcluster, "output cluster"=w422:T11, "VISA resource name out"=w438:refnum<visa-resource-name>)  [unwired: 6 in]
              n149 = call "MDAQ_CursorHelp.vi"("Input Cluster"=w422) -> ("X-Cursor-1"=w417:dbl, "X-Cursor-0"=w419:dbl)  [unwired: 9 in]
              n150 = call "MDAQ_READ_Spectrum.vi"("error in"=w437, "Status_Cluster IN"=w422, "Mode"=enum16{"ASCII"}."ASCII", "VISA resource name"=w438) -> ("error out"=w431:errorcluster, "output cluster"=w411:T11, "Output Array"=w412:u32[], "VISA resource name out"=w432:refnum<visa-resource-name>)  [unwired: 4 in]
              "CurrectSpectrum" <- w412
              n151 = property class="WFGraph (strict)"(reference=w421, "Active Cursor"=u32 0, "Cursor.Cursor X"=w419, "Active Cursor"=u32 1, "Cursor.Cursor X"=w417) -> ()  [unwired: 1 in, 2 out]
              n152 = call "MDAQ_READ_Sum.vi"("error in"=w431, "VISA resource name"=w432) -> ("error out"=w425:errorcluster, "Sum"=w428:u32, "VISA resource name out"=w426:refnum<visa-resource-name>)  [unwired: 7 in]
              n153 = case shown="\"CV+Temp\"" w430 {
                tunnel: [Status_Def."Idle" ("Enum") Status_Def."ConfigCV" ("Enum") Status_Def."ConfigCV" ("Enum")] -> w429
                tunnel: w428 -> [_ w447 w454]
                tunnel: w427 -> [w440 w446 w453]
                tunnel: [w440 w444 w451] -> w410
                tunnel: [w439 w442 w450] -> w401
                tunnel: w402 -> [w439 w443 w449]
                frame "Off", Default {
                }
                frame "CV" {
                  n154 = call "MDAQ_ArrayHelp.vi"("Sum"=w447, "Input Cluster"=w446, "Concurrent CV Arrays"=w443) -> ("Output Cluster"=w445:T12, "Concurrent CV Arrays Out"=w442:T10)  [unwired: 7 in]
                  n155 = call "MDAQ_IndexInc.vi"("Input Cluster"=w445) -> ("Output Cluster"=w444:T12)  [unwired: 10 in]
                }
                frame "CV+Temp" {
                  n156 = call "MDAQ_ArrayHelp.vi"("Sum"=w454, "Input Cluster"=w453, "Concurrent CV Arrays"=w449) -> ("Output Cluster"=w452:T12, "Concurrent CV Arrays Out"=w450:T10)  [unwired: 7 in]
                  n157 = call "MDAQ_IndexInc.vi"("Input Cluster"=w452) -> ("Output Cluster"=w451:T12)  [unwired: 10 in]
                }
              }
              n158 = control-ref of="Amplitude Plot"() -> (w404:refnum<vi>)
              n159 = Unbundle By Name(w410) -> ("CV.CycleNo"=→"Current Scan No.":i32)
              n160 = call "MDAQ_CollectSurfaceSpectrum.vi"("Cluster IN"=w410, "Status Cluster In"=w411, "CurrectSpectrum"=w412) -> ("Cluster Out"=w408:T12, "Status Cluster Out"=w409:T11)  [unwired: 7 in]
              n161 = call "MDAQ_GraphHelper.vi"("Concurrent CV Arrays"=w401, "Normalised"="Normalise Graph", "Input Cluster"=w410, "Amplitude Plot"=w404) -> ("To Temp Graph"=→"Temp Graph":T4, "To Graph"=→"XY Graph":T3, "Array"=→"Amplitude Plot":cluster{"Numeric":dbl, dbl}[])  [unwired: 5 in]
              n162 = call "MDAQ_SurfaceSum.vi"("Cluster IN"=w408, "Status_Cluster IN"=w409) -> ("Cluster Out"=w406:T12, "Status_Cluster Out"=w407:T11, "CV.SurfaceCV"=→"Surface CV Plot":dbl[][])  [unwired: 7 in]
              n163 = call "MDAQ_ClearSpec.vi"("error in (no error)"=w425, "VISA Refnum in"=w426) -> ("error out"=w423:errorcluster, "VISA Refnum out"=w424:refnum<visa-resource-name>)  [unwired: 8 in]
            }
            frame "RefreshCV" {
              n164 = control-ref of="Normalise Graph"() -> (w464:refnum<vi>)
              n165 = control-ref of="XY Graph"() -> (w463:refnum<vi>)
              n166 = control-ref of="Target Bins/Ampl"() -> (w473:refnum<vi>)
              n167 = control-ref of="Delta T (s)"() -> (w471:refnum<vi>)
              n168 = property class="DigNum (strict)"(reference=w471) -> ("Value"=w469:dbl)  [unwired: 1 in, 2 out]
              n169 = property class="Arr (strict)"(reference=w473) -> ("Value"=w472:dbl[])  [unwired: 1 in, 2 out]
              n170 = property class="Bool (strict)"(reference=w464) -> ("Value"=w461:bool)  [unwired: 1 in, 2 out]
              n171 = Array Size(array="Target Bins/Ampl") -> (size(s)=w465:i32)
              n172 = Array Size(array=w472) -> (size(s)=w470:i32)
              "Target Values" <- w470
              n173 = shared-variable ".\\VariableLib.lvlib\\Connected"(error in=w458) -> (→"LakeShore?":bool, error out=w457:errorcluster)
              n174 = Bundle By Name(cluster=w467, "CV.Target Set Points"="Target Bins/Ampl", "CV.No. Set Points"=w465) -> (w462:T12)
              n175 = Multiply(x=w470, y=w469) -> (x*y=→"Delta T per Cycle (s)":dbl)
              n176 = control-ref of="Amplitude Plot"() -> (w460:refnum<vi>)
              n177 = call "MDAQ_CVPlotHelper.vi"("Amplitude Plot"=w460, "Normalised"=w461, "Input Cluster"=w462, "XY Graph ref"=w463) -> ()  [unwired: 8 in]
            }
            frame "Read Help" {
              n178 = call "MDAQ_WRITE.vi"("error in"=w487, "ARG"="", "CMD"="H" ("write buffer"), "VISA resource name"=w488) -> ("error out"=w486:errorcluster, "VISA resource name out"=w485:refnum<visa-resource-name>)  [unwired: 6 in]
              n179 = Bundle By Name(cluster=w483, "Request Read"=TRUE) -> (w481:T12)
            }
            frame "Clear Monitor" {
              n180 = Bundle By Name(cluster=w496, "Request Read"=FALSE, "Monitor MSG"="") -> (w494:T12)
            }
            frame "Settings Send" {
              n181 = Bundle By Name(cluster=T15 {"Freq"=0.0, "Amp"=0.0, "Chan Start"=0.0, "Chan End"=0.0, "Wave Form"=enum."Item 0", "Channels"=enum."Item 0"} ("ARG Cluster"), "Freq"="Frequency", "Amp"="Amplitude", "Chan Start"="Gate Start", "Chan End"="Gate Stop", "Wave Form"="Wave Form", "Channels"="Channels") -> (w506:T15)
              n182 = call "MDAQ_Settings_Set.vi"("error in"=w499, "Status_Cluster"=w500, "ARG Cluster"=w506, "VISA resource name"=w501) -> ("error out"=w504:errorcluster, "Status_Cluster Out"=w503:T11, "VISA resource name out"=w505:refnum<visa-resource-name>)  [unwired: 5 in]
              n183 = Bundle By Name(cluster=w515, "Request Read"=TRUE) -> (w514:T12)
            }
            frame "Get Spectrum" {
              n184 = control-ref of="Waveform Graph"() -> (w523:refnum<vi>)
              n185 = Unbundle By Name(w526) -> ("Getting Mode"=w525:T13)
              n186 = call "MDAQ_READ_Status.vi"("error in"=w535, "Status_Cluster IN"=w534, "VISA resource name"=w536) -> ("error out"=w530:errorcluster, "output cluster"=w522:T11, "VISA resource name out"=w531:refnum<visa-resource-name>)  [unwired: 6 in]
              n187 = case shown="\"Normal\"" w525 {
                tunnel: [Status_Def."Idle" ("Enum") Status_Def."StartAq" ("t")] -> w524
                frame "Off", Default {
                }
                frame "Normal" {
                }
              }
              n188 = call "MDAQ_READ_Spectrum.vi"("error in"=w530, "Status_Cluster IN"=w522, "Mode"=enum16{"ASCII"}."ASCII", "VISA resource name"=w531) -> ("error out"=w527:errorcluster, "output cluster"=w521:T11, "Output Array"=w520:u32[], "VISA resource name out"=w528:refnum<visa-resource-name>)  [unwired: 4 in]
              n189 = call "MDAQ_GraphCursors.vi"("Status Cluster"=w521, "Input Array"=w520, "Graph Ref"=w523) -> ("Status Cluster Out"=w519:T11, "Output Array"=→"Waveform Graph":u32[])  [unwired: 7 in]
              n190 = Bundle By Name(cluster=w526, "Request Read"=FALSE) -> (w533:T12)
            }
            frame "SaveSpectrum" {
              n191 = Unbundle By Name(w541) -> ("Spectrum Array"=w540:u32[])
              n192 = Unbundle By Name(w549) -> ("Normal.Collecting"=w548:bool)
              n193 = Select(t=Status_Def."StartAq", s=w548, f=Status_Def."Idle" ("Enum")) -> (s? t:f=w545:T9)
              n194 = call "MDAQ_SaveSpectrum.vi"("error in"=w542, "Input Array"=w540) -> ("error out"=w544:errorcluster)  [unwired: 9 in]
              n195 = Bundle By Name(cluster=w549, "Request Read"=FALSE) -> (w551:T12)
            }
            frame "LoadSpectrum" {
              n196 = control-ref of="Waveform Graph"() -> (w554:refnum<vi>)
              n197 = call "MDAQ_SpectrumLoad.vi"("error in"=w557, "Status_Cluster"=w558) -> ("error IO"=w556:errorcluster, "Status_Cluster Out"=w555:T11)  [unwired: 8 in]
              n198 = Unbundle By Name(w555) -> ("Spectrum Array"=w553:u32[])
              n199 = property class="WFGraph (strict)"(reference=w554, "Value"=w553) -> ()  [unwired: 1 in, 2 out]
            }
            frame "SaveCVPlot" {
              n200 = call "MDAQ_SaveCVFile.vi"("error in"=w563, "Control Cluster"=w564, "Concurrent CV Arrays"=w562) -> ("error out"=w565:errorcluster)  [unwired: 8 in]
            }
            frame "WriteCVData" {
              n201 = call "MDAQ_SaveCVSpectrums.vi"("User Comment"="User Comments", "Sample Name"="Sample Name", "error in"=w577, "Control Cluster"=w575, "Status_Cluster"=w576, "file path (use dialog)"="Master File Path") -> ("error out"=w574:errorcluster, "Control Cluster Out"=w571:T12, "Status_Cluster Out"=w572:T11)  [unwired: 3 in]
            }
            frame "ClearCVCycle" {
              n202 = in-place {
                n203 = in-place-cluster #1(w583) -> ("Spectrum Cycle"=w590:u32[][])
                n204 = in-place-cluster #2(w585) -> ()  [unwired: 1 out]
                n205 = for {
                  tunnel: w590 -> [w593] mode=indexing
                  tunnel: [w592] -> w589 mode=indexing
                  n206 = for {
                    tunnel: w593 -> [_] mode=indexing
                    tunnel: [u32 0] -> w592 mode=indexing
                  }
                }
                n207 = in-place-cluster #1("Spectrum Cycle"=w589) -> (w582:T11)
                n208 = in-place-cluster #2("CV.New Cycle"=FALSE) -> (w584:T12)
              }
            }
          }
          n209 = Unbundle By Name(w104) -> ("Monitor MSG"=→"MDAQ Monitor":string)
          n210 = call "MDAQ_MsgCuller.vi"("Main Cluster"=w104) -> ("Main Out"=w103:T12)  [unwired: 10 in]
          n211 = Or(x=w116, y=w115) -> (x .or. y?=w114:bool)
          n212 = Wait (ms)(milliseconds to wait=u32 30) -> ()  [unwired: 1 out]
        }
      }
      frame Error {
      }
    }
  }
  n213 = control-ref of="StopAq_Button"() -> (w1:refnum<vi>)
  n214 = control-ref of="StartAq_Button"() -> (w2:refnum<vi>)
  n215 = property class="Bool"(reference=w2, "DisabledEnum"=T8."Enabled" ("Disabled")) -> ()  [unwired: 1 in, 2 out]
  n216 = property class="Bool"(reference=w1, "DisabledEnum"=T8."Disabled and Grayed Out" ("Disabled")) -> ()  [unwired: 1 in, 2 out]
  n217 = VISA Close(VISA resource name=w8, error in (no error)=w7) -> (error out=→"error out":errorcluster)
